vi "toBoolNotifier.vi"(8 "error in":errorcluster, 11 "ITaskChannel":refnum<class "ITaskChannel.lvclass">) -> (0 "error out":errorcluster, 3 "boolNotifier":refnum<notifier>)   [LabVIEW 2023, in "TLC_Daemon.lvlib"]
uses:
  TLC_Daemon.lvlib
  ITaskChannel/ITaskChannel.lvclass
  BoolNotifierTaskChannel/BoolNotifierTaskChannel.lvclass
  BoolNotifierTaskChannel/BoolNotifierTaskChannel.lvclass/BoolNotifierTaskChannel.ctl
  NotifierStopMechanism/Read notifierRef.vi
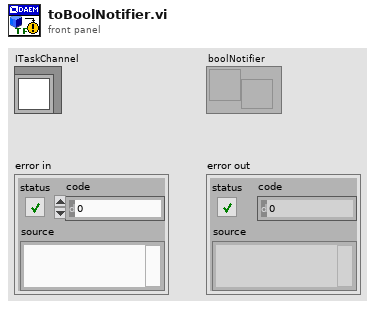
[diagram p1: front panel]
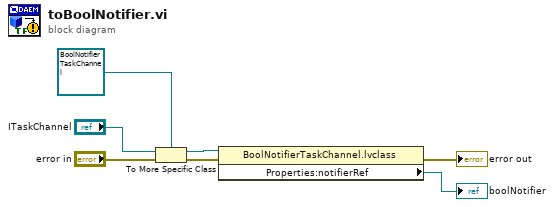
[diagram p0: block diagram]
diagram:
  n1 = To More Specific Class(target class=refnum<class "BoolNotifierTaskChannel.lvclass"> refnum ("TLC_Daemon.lvlib:NotifierStopMechanism.lvclass"), reference="ITaskChannel", error in="error in") -> (specific class reference=w4:refnum<class "BoolNotifierTaskChannel.lvclass">, error out=w6:errorcluster)
  n2 = property class="BoolNotifierTaskChannel.lvclass"(reference=w4, error in=w6) -> (error out=→"error out":errorcluster, "Properties:notifierRef"=→"boolNotifier":refnum<notifier>)  [unwired: 1 out]
